vi "Add Hardware.vi"(0 "Microscope in":refnum<class "Microscope.lvclass">, 5 "Device.lvlib:Device.lvclass":refnum<class "Device.lvclass">, 7 "Label":string, 11 "error in (no error)":errorcluster) -> (4 "Microscope out":refnum<class "Microscope.lvclass">, 6 "Nested Actor's Enqueuer":refnum<class "Message Enqueuer.lvclass">, 8 "key already included?":bool, 10 "value unchanged?":bool, 15 "error out":errorcluster)   [LabVIEW 2020, in "Microscope.lvlib" / "Microscope.lvclass"]
uses:
  Microscope.lvclass
  C:/Program Files/National Instruments/LabVIEW 2020/vi.lib/ActorFramework/Actor/Actor.lvclass
  Component/Device/Device/Device.lvclass
  <vilib>/ActorFramework/Message Enqueuer/Message Enqueuer.lvclass
  Microscope.lvclass/Microscope.ctl
  <vilib>/ActorFramework/Actor/Actor.lvclass
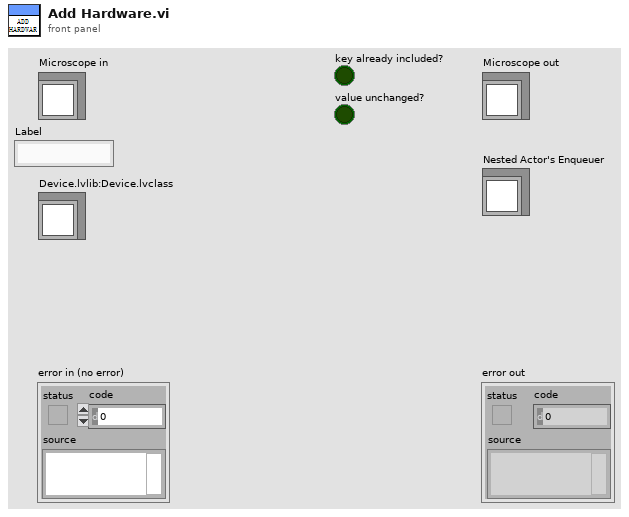
[diagram p1: front panel]
types:
  T1 = map{string, refnum<class "Message Enqueuer.lvclass">}
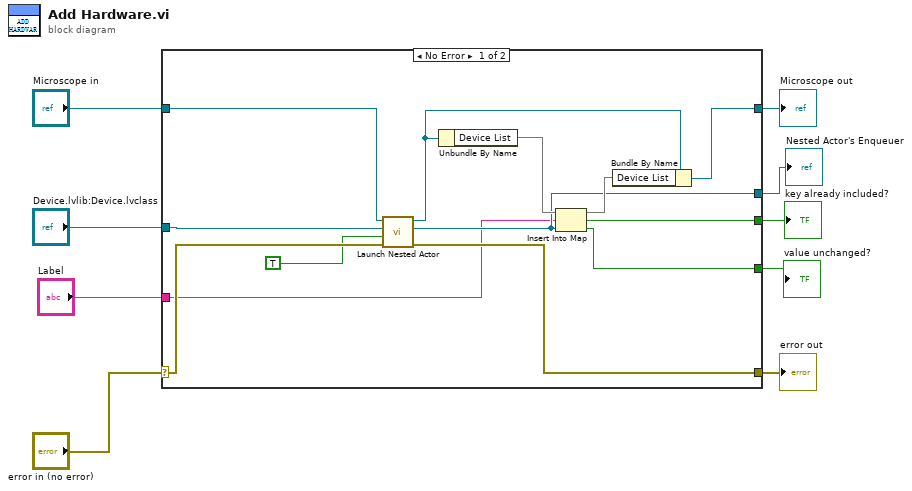
[diagram p0: block diagram]
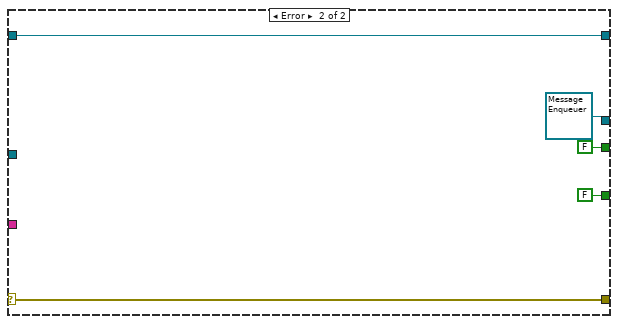
[diagram p2: hidden frame]
diagram:
  n1 = case shown="No Error" "error in (no error)" {
    selector: "error in (no error)" -> [w13 w27]
    tunnel: [w15 w27] -> w8
    tunnel: [w16 w26] -> w6
    tunnel: "Microscope in" -> [w22 w26]
    tunnel: "Device.lvlib:Device.lvclass" -> [w12 _]
    tunnel: [w18 FALSE ("key already included?")] -> w4
    tunnel: [w17 FALSE ("value unchanged?")] -> w3
    tunnel: [w14 refnum<class "Message Enqueuer.lvclass"> refnum ("Nested Actor's Enqueuer")] -> w2
    tunnel: "Label" -> [w11 _]
    frame No Error {
      n2 = call <vilib>:"Launch Nested Actor.vi"("error in (no error)"=w13, "Auto-stop? (T)"=TRUE, "Nested Actor"=w12, "Caller Actor in"=w22) -> ("error out"=w15:errorcluster, "Nested Actor's Enqueuer"=w14:refnum<class "Message Enqueuer.lvclass">, "Caller Actor out"=w20:refnum<class "Microscope.lvclass">)  [unwired: 5 in]
      n3 = Unbundle By Name(w20) -> ("Device List"=w21:T1)
      n4 = Insert Into Map(map in=w21, key=w11, value=w14) -> (map out=w19:T1, key already included?=w18:bool, value unchanged?=w17:bool)
      n5 = Bundle By Name(cluster=w20, "Device List"=w19) -> (w16:refnum<class "Microscope.lvclass">)
    }
    frame Error {
    }
  }
  "error out" <- w8
  "Microscope out" <- w6
  "key already included?" <- w4
  "value unchanged?" <- w3
  "Nested Actor's Enqueuer" <- w2
